vi "setShowCursors.vi"(8 "error in (no error)":errorcluster, 10 "Visible":bool, 11 "QControl_Graph in":refnum<class "QControl_Graph.lvclass">) -> (0 "error out":errorcluster, 3 "QControl_Graph out":refnum<class "QControl_Graph.lvclass">)   [LabVIEW 2017, in "QControl_Graph.lvclass"]
uses:
  QControl_Graph.lvclass
  QControl_Graph.lvclass/QControl_Graph.ctl
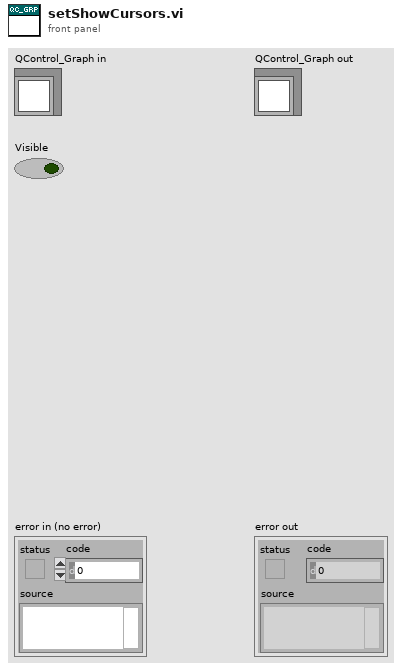
[diagram p1: front panel]
types:
  T1 = typedef "QControl_Graph.lvclass/State Data.ctl" = cluster{"Action Performed":refnum<user-event>, "Show Cursors":bool, "Cursor Properties":T2}
  T2 = typedef "QControl_Graph.lvclass/Cursor Properties.ctl" = cluster{"Horizontal Line?":bool, "Vertical Line?":bool, "Timestamp":enum16{"at TOP", "at BOTTOM", "none"}, "time format (%H:%M:%S)":string, "size":i16, "font":T3, "alignment(left, top)":T4, "TextFormat":string}
  T3 = typedef "QControl_Graph.lvclass/Font.ctl" = cluster{"Font Name":string, "Size":i16, "Strikeout?":bool, "Italic?":bool, "Underline?":bool, "Outline?":bool, "Shadow":bool, "Bold?":bool}
  T4 = typedef "QControl_Graph.lvclass/Alignment.ctl" = cluster{"Horizontal":T5, "Vertical":T6}
  T5 = typedef "QControl_Graph.lvclass/Alignment.Horizontal.ctl" = enum16{"left", "center", "right"}
  T6 = typedef "QControl_Graph.lvclass/Alignment.Vertical.ctl" = enum16{"top", "center", "bottom"}
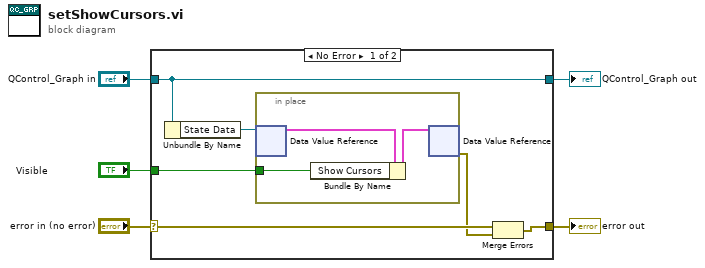
[diagram p0: block diagram]
diagram:
  n1 = case shown="No Error" "error in (no error)" {
    selector: "error in (no error)" -> [w11 w16]
    tunnel: [w8 w16] -> w3
    tunnel: [w10 w15] -> w2
    tunnel: "QControl_Graph in" -> [w10 w15]
    tunnel: "Visible" -> [w6 _]
    frame No Error {
      n2 = Unbundle By Name(w10) -> ("State Data"=w9:refnum<data-value>)
      n3 = in-place {
        in-place-border: w6 -> [w12]
        n4 = in-place-dvr #1(w9) -> (w14:T1)  [unwired: 1 out]
        n5 = Bundle By Name(cluster=w14, "Show Cursors"=w12) -> (w13:T1)
        n6 = in-place-dvr #1(w13) -> (w7:errorcluster)  [unwired: 1 out]
      }
      n7 = Merge Errors(w11, w7) -> (w8:errorcluster)
    }
    frame Error {
    }
  }
  "error out" <- w3
  "QControl_Graph out" <- w2
